vi "Basic LabVIEW OPC UA Client-Write.vi"() -> ()   [LabVIEW 2020]
uses:
  <vilib>/OPCUA/controls/NodeId.ctl
  <vilib>/OPCUA/controls/Write Status.ctl
  <vilib>/OPCUA/client/Multiple Write Double.vi
  <vilib>/OPCUA/NI OPC UA Client.lvlib
  <vilib>/OPCUA/NI OPC UA Utility.lvlib
panel:
  in  "Item Path":string="Nodes.Temperature"
  in  "Stop Button":bool
  in  "Temperature Value":dbl=23.0
  in  "Server Endpoint URL":string="opc.tcp://XPS15HPH:49580"
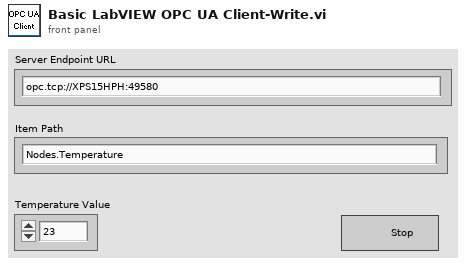
[diagram p1: front panel]
types:
  T1 = cluster{"message mode":enum16{"None", "Sign", "Sign and Encrypt"}, "security":enum16{"Basic256", "Basic128Rsa15"}}
  T2 = typedef "OPC UA Client Refnum.ctl" = refnum<k21>
  T3 = typedef "NodeId.ctl" = string
  T4 = typedef "Write Status.ctl" = u32
  T5 = cluster{"node ID":T3, "value":dbl, "timestamp (current time)":timestamp, "node status":T4}
  T6 = cluster{"node ID":T3, "value":dbl, "timestamp (current time)":timestamp, "node status":T4}[]
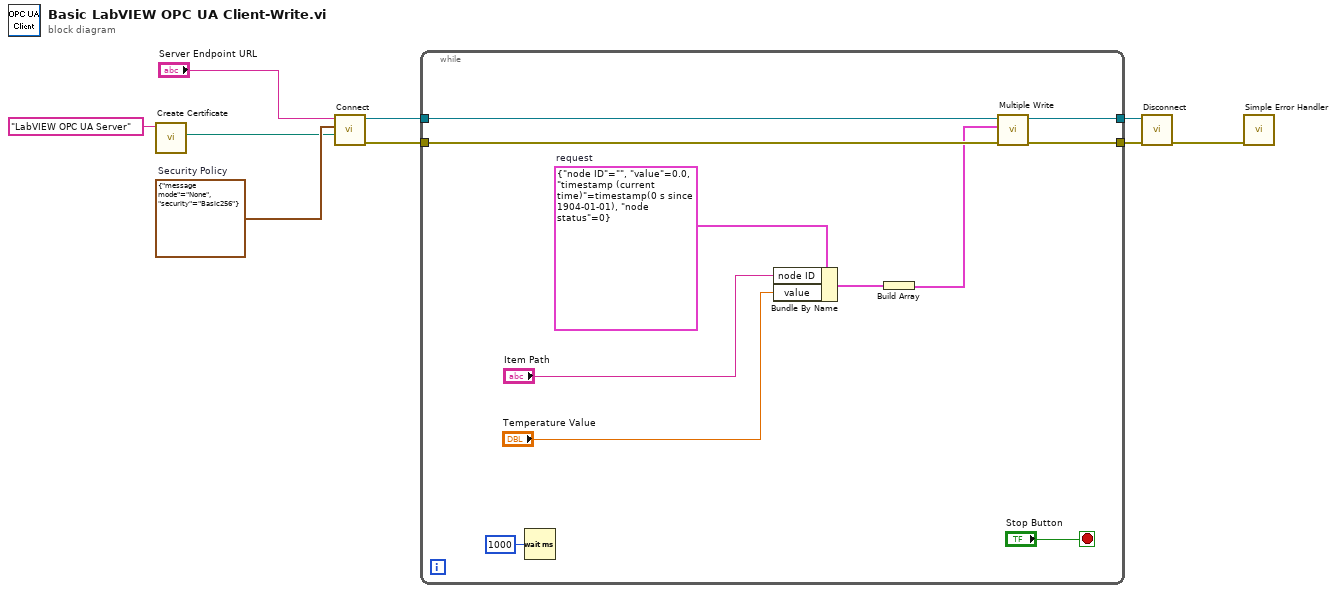
[diagram p0: block diagram]
diagram:
  w3 = T1 {"message mode"=enum."None", "security"=enum."Basic256"}  # Security Policy
  n1 = call <vilib>:"Create Certificate.vi"("certificate name in"="LabVIEW OPC UA Server") -> ("certificate path"=w1:path)  [unwired: 7 in, 3 out]
  n2 = call <vilib>:"Connect.vi"("client certificate file"=w1, "security policy"=w3, "server endpoint URL"="Server Endpoint URL") -> ("error out"=w8:errorcluster, "OPC UA client refnum out"=w9:T2)  [unwired: 6 in, 1 out]
  n3 = while {
    tunnel: w9 -> [w18]
    tunnel: w8 -> [w17]
    tunnel: [w16] -> w7
    tunnel: [w15] -> w5
    stop <- "Stop Button" stop-if-true
    w14 = T5 {"node ID"="", "value"=0.0, "timestamp (current time)"=timestamp(0 s since 1904-01-01), "node status"=0}  # request
    n4 = Wait (ms)(milliseconds to wait=u32 1000) -> ()  [unwired: 1 out]
    n5 = Bundle By Name "Bundle By Name"(cluster=w14, "node ID"="Item Path", "value"="Temperature Value") -> (w10:T5)
    n6 = Build Array "Build Array"(w10) -> (w11:T6)
    n7 = call-poly <vilib>:"Multiple Write.vi"("error in (no error)"=w17, "requests"=w11, "OPC UA client refnum in"=w18) -> ("error out"=w15:errorcluster, "OPC UA client refnum out"=w16:T2)  [unwired: 5 in, 2 out]
  }
  n8 = call <vilib>:"Disconnect.vi"("error in (no error)"=w5, "OPC UA client refnum in"=w7) -> ("error out"=w6:errorcluster)  [unwired: 9 in]
  n9 = call <vilib>:"Simple Error Handler.vi"("error in (no error)"=w6) -> ()  [unwired: 4 in, 5 out]
